vi "Demo Accelerometer Graph.vi"(8 "error in (no error)":errorcluster) -> (0 "error out":errorcluster)   [LabVIEW 2011]
uses:
  VIremote.llb/VIremoteEvent.ctl
  VIremote.llb/VIremoteFunction.ctl
panel:
  in  "VIremoteEvent":T1=enum."Connection Closed"
  out "Waveform Chart":cluster{"X":dbl, "Y":dbl, "Z":dbl}(graph)
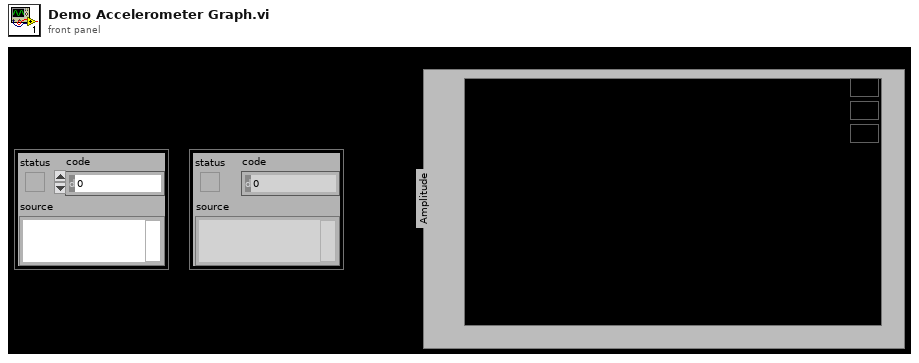
[diagram p1: front panel]
types:
  T1 = typedef "VIremoteEvent.ctl" = enum16{"No Event", "Connection Closed", "Navigate Back", "Enter Background", "Enter Foreground", "Portrait", "Portrait Upside Down", "Landscape Left", "Landscape Right"}
  T2 = typedef "VIremoteFunction.ctl" = enum16{"Do nothing", "Stop controller", "Close this connection", "Show info panel", "Set VI to control", "Set Accelerometer freq (Hz)", "Show Alert message", "Start Sound Input", "Stop Sound Input", "Set Volume (0-100)", "Set sound output Speaker", "Set sound output Receiver", "Play Sound", "Repeat Sound", "Stop Sound", "Pause Sound", "Resume Sound", "Set panel width of caller (320 or 480)", "Set Panel Size to Portrait", "Set Panel Size to Landscape", "Set Panel Size as Current Orientation", "Allow all UI Orientations", "Send user notification", "Disable Scrolling", "Normal Scrolling", "Page Scrolling", "Set Scroll Offset", "Page Indicator Position"}
  T3 = cluster{"UIorientation":refnum<notifier>, "Accelerometer":refnum<notifier>, "Sound":refnum<notifier>, "SoundPlayBufferReady":refnum<notifier>, "BackgroundState":refnum<notifier>, "Touch":refnum<notifier>}
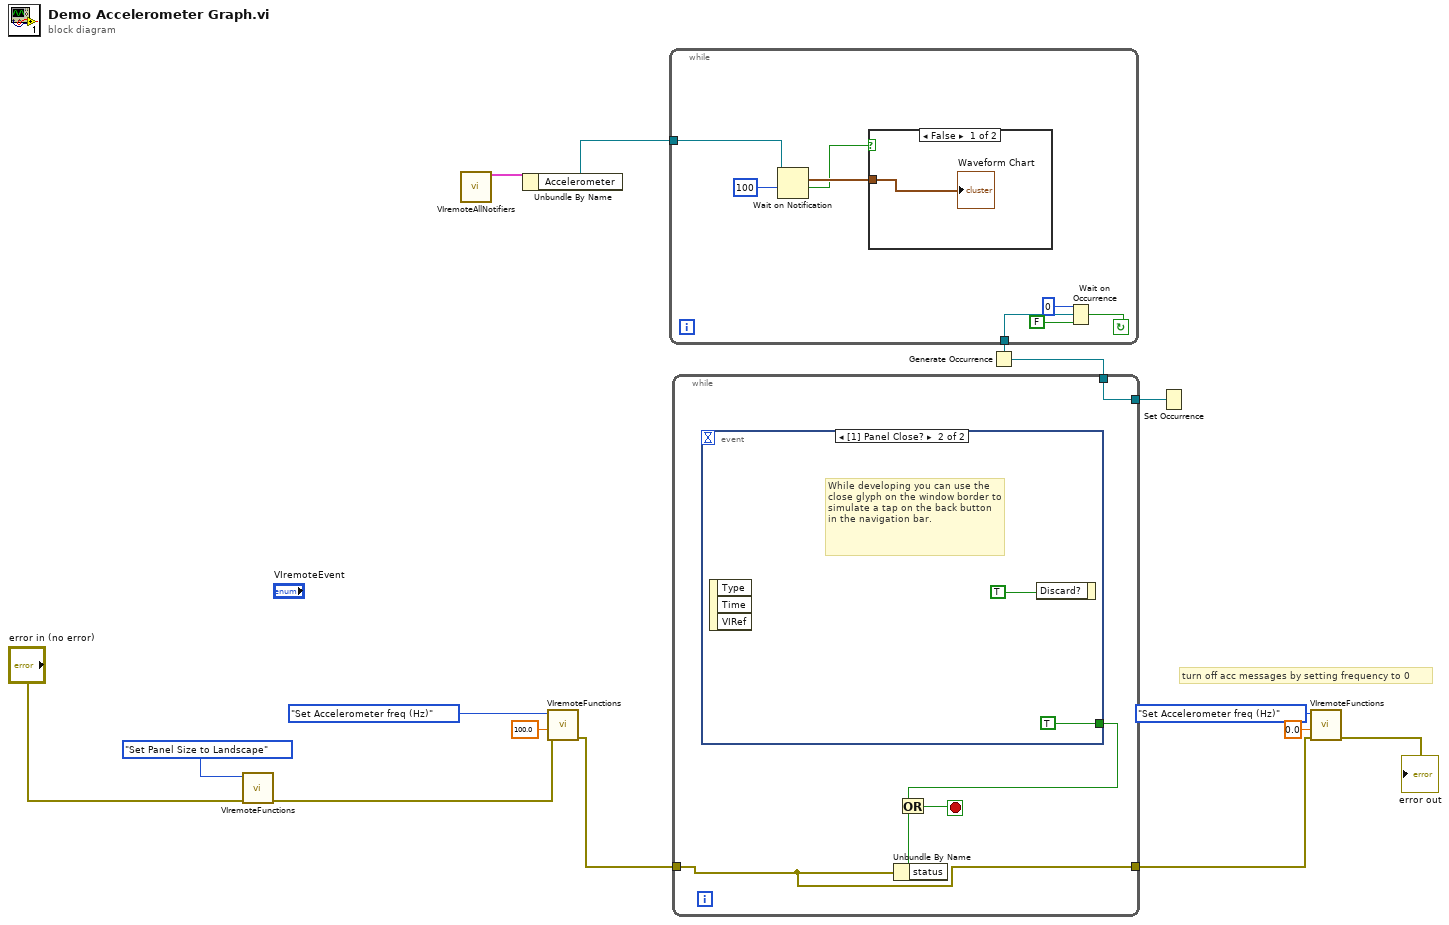
[diagram p0: block diagram]
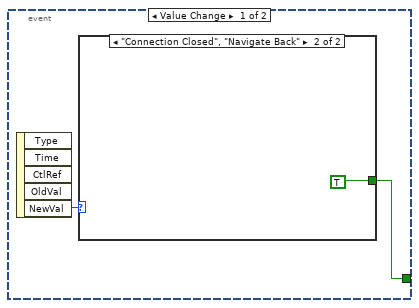
[diagram p3: hidden frame]
diagram:
  # "turn off acc messages by setting frequency to 0"
  n1 = call "VIremoteFunctions.vi"("error in (no error)"="error in (no error)", "Function"=VIremoteFunction."Set Panel Size to Landscape") -> ("error out"=w7:errorcluster)  [unwired: 4 in, 5 out]
  n2 = call "VIremoteAllNotifiers.vi"() -> ("All Notifiers (unbundle by name)"=w4:T3)  [unwired: 1 in, 10 out]
  n3 = Unbundle By Name(w4) -> ("Accelerometer"=w3:refnum<notifier>)
  n4 = call "VIremoteFunctions.vi"("error in (no error)"=w7, "Value in"=100.0, "Function"=VIremoteFunction."Set Accelerometer freq (Hz)") -> ("error out"=w12:errorcluster)  [unwired: 3 in, 5 out]
  n5 = Generate Occurrence() -> (w1:refnum<k4>)
  n6 = while {
    tunnel: w3 -> [w21]
    tunnel: w1 -> [w20]
    stop <- w17 continue-if-true
    n7 = Wait on Notification(notifier=w21, timeout in ms (-1)=100) -> (notification=w22:cluster{"X":dbl, "Y":dbl, "Z":dbl}, timed out?=w15:bool)  [unwired: 1 in, 3 out]
    n8 = case shown="False" w15 {
      tunnel: w22 -> [w23 _]
      frame False {
        "Waveform Chart" <- w23
      }
      frame True {
        # "Timeout"
      }
    }
    n9 = Wait on Occurrence(1:FALSE ("ignore previous (T)"), 2:w20, 3:0 ("ms timeout (-1)")) -> (0:w17:bool)
  }
  n10 = while {
    tunnel: w12 -> [w26]
    tunnel: [w26] -> w9
    tunnel: w1 -> [w24]
    tunnel: [w24] -> w2
    stop <- w27 stop-if-true
    n11 = event shown="[1] Panel Close?" {
      selector: _ -> [_ _]
      dyn-events: _ -> [_ _]
      timeout: _ -> [_ _]
      tunnel: [w30 TRUE ("Discard?")] -> w25
      event Value Change {
        n12 = event-data() -> ("NewVal"=w29:T1)  [unwired: 5 out]
        n13 = case shown="\"Connection Closed\", \"Navigate Back\"" w29 {
          tunnel: [_ TRUE] -> w30
          frame "No Event", Default {
          }
          frame "Connection Closed", "Navigate Back" {
          }
        }
      }
      event Panel Close? {
        # "While developing you can use the close glyph on the window border to simulate a tap on the back button in the navigation bar."
        n14 = event-data() -> ()  [unwired: 4 out]
        n15 = event-data("Discard?"=TRUE) -> ()  [unwired: 1 in, 1 out]
      }
    }
    n16 = Unbundle By Name(w26) -> ("status"=w28:bool)
    n17 = Or(x=w25, y=w28) -> (x .or. y?=w27:bool)
  }
  n18 = Set Occurrence(w2) -> ()
  n19 = call "VIremoteFunctions.vi"("error in (no error)"=w9, "Value in"=0.0, "Function"=VIremoteFunction."Set Accelerometer freq (Hz)") -> ("error out"=→"error out":errorcluster)  [unwired: 3 in, 5 out]
